vi "周期设置_氨氮.vi"() -> ()   [LabVIEW 2016, in "斯坦道氨氮.lvlib"]
uses:
  <vilib>/Utility/miscctls.llb/LVPointTypeDef.ctl
  <vilib>/Utility/config.llb/NI_LVConfig.lvlib
panel:
  in  "运行周期":T1={"运行模式"=enum."维护模式", "质控频次"=enum."关闭", "空白核查时间"=2, "跨度核查时间"=6, "24H周期设置"=[]} {"跨度核查时间" items=["00H", "01H", "02H", "03H", "04H", "05H", "06H", "07H", "08H", "09H", "10H", "11H", "12H", "13H", "14H", "15H", "16H", "17H", "18H", "19H", "20H", "21H", "22H", "23H", "关闭"]; "空白核查时间" items=["00H", "01H", "02H", "03H", "04H", "05H", "06H", "07H", "08H", "09H", "10H", "11H", "12H", "13H", "14H", "15H", "16H", "17H", "18H", "19H", "20H", "21H", "22H", "23H", "关闭"]}
  # "运行模式："
  # "质控频次："
  # "零点核查时间："
  # "跨度核查时间："
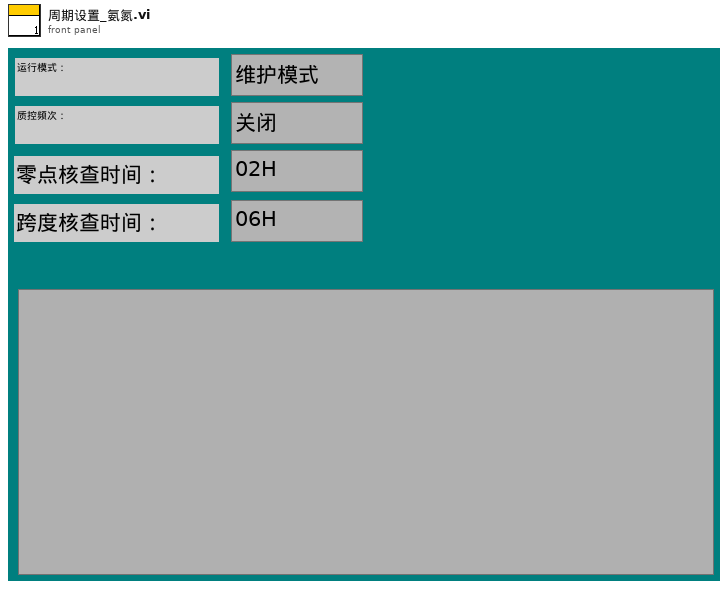
[diagram p1: front panel]
types:
  T1 = cluster{"运行模式":enum16{"维护模式", "常规模式", "应急模式", "质控模式"}, "质控频次":enum16{"关闭", "每天", "星期一", "星期二", "星期三", "星期四", "星期五", "星期六", "星期日"}, "空白核查时间":u16, "跨度核查时间":u16, "24H周期设置":bool[]}
  T2 = typedef "LVPointTypeDef.ctl" = cluster{"Horizontal":i16, "Vertical":i16}
  T3 = enum16{"启动测量", "标样核查", "零点核查", "跨度核查", "空白测试", "平行样测试", "加标回收", "空白校准", "标样校准", "初始化（清洗）", "停止测试", "仪器重启", "校时", "模式设置", "测量间隔设置"}
  T4 = cluster{"系统时间":timestamp, "工作状态":enum16{"空闲", "水样测试", "标样核查", "零点核查", "跨度核查", "空白测试", "平行样测试", "加标回收", "空白校准", "标样校准", "初始化（清洗）"}, "测量模式":enum16{"待机", "连续模式", "周期模式", "定点模式", "受控模式", "手动模式"}, "告警代码":u16, "故障代码":u16, "日志代码":u16, "软件版本":u16, "F0":sgl, "F1":sgl, "F2":sgl, "F3":sgl, "T":sgl, "H":sgl, "id":u16, "flowid":u16, "量程":u16, "总磷控温温度1":sgl, "营养盐控温温度2":sgl, "ADC":sgl}
  T5 = enum16{"关闭", "每天", "星期一", "星期二", "星期三", "星期四", "星期五", "星期六", "星期日"}
  T6 = typedef "LVDateTimeRec.ctl" = cluster{"秒数的小数部分":dbl, "秒":i32, "分":i32, "时":i32, "日":i32, "月":i32, "年":i32, "天数（周）":i32, "天数（年）":i32, "DST":i32}
  T7 = enum32{"Bad", "Idle", "Run top level", "Running"}
  T8 = typedef "NI_LVConfig.lvlib/Config Data RefNum.ctl" = refnum<k1>
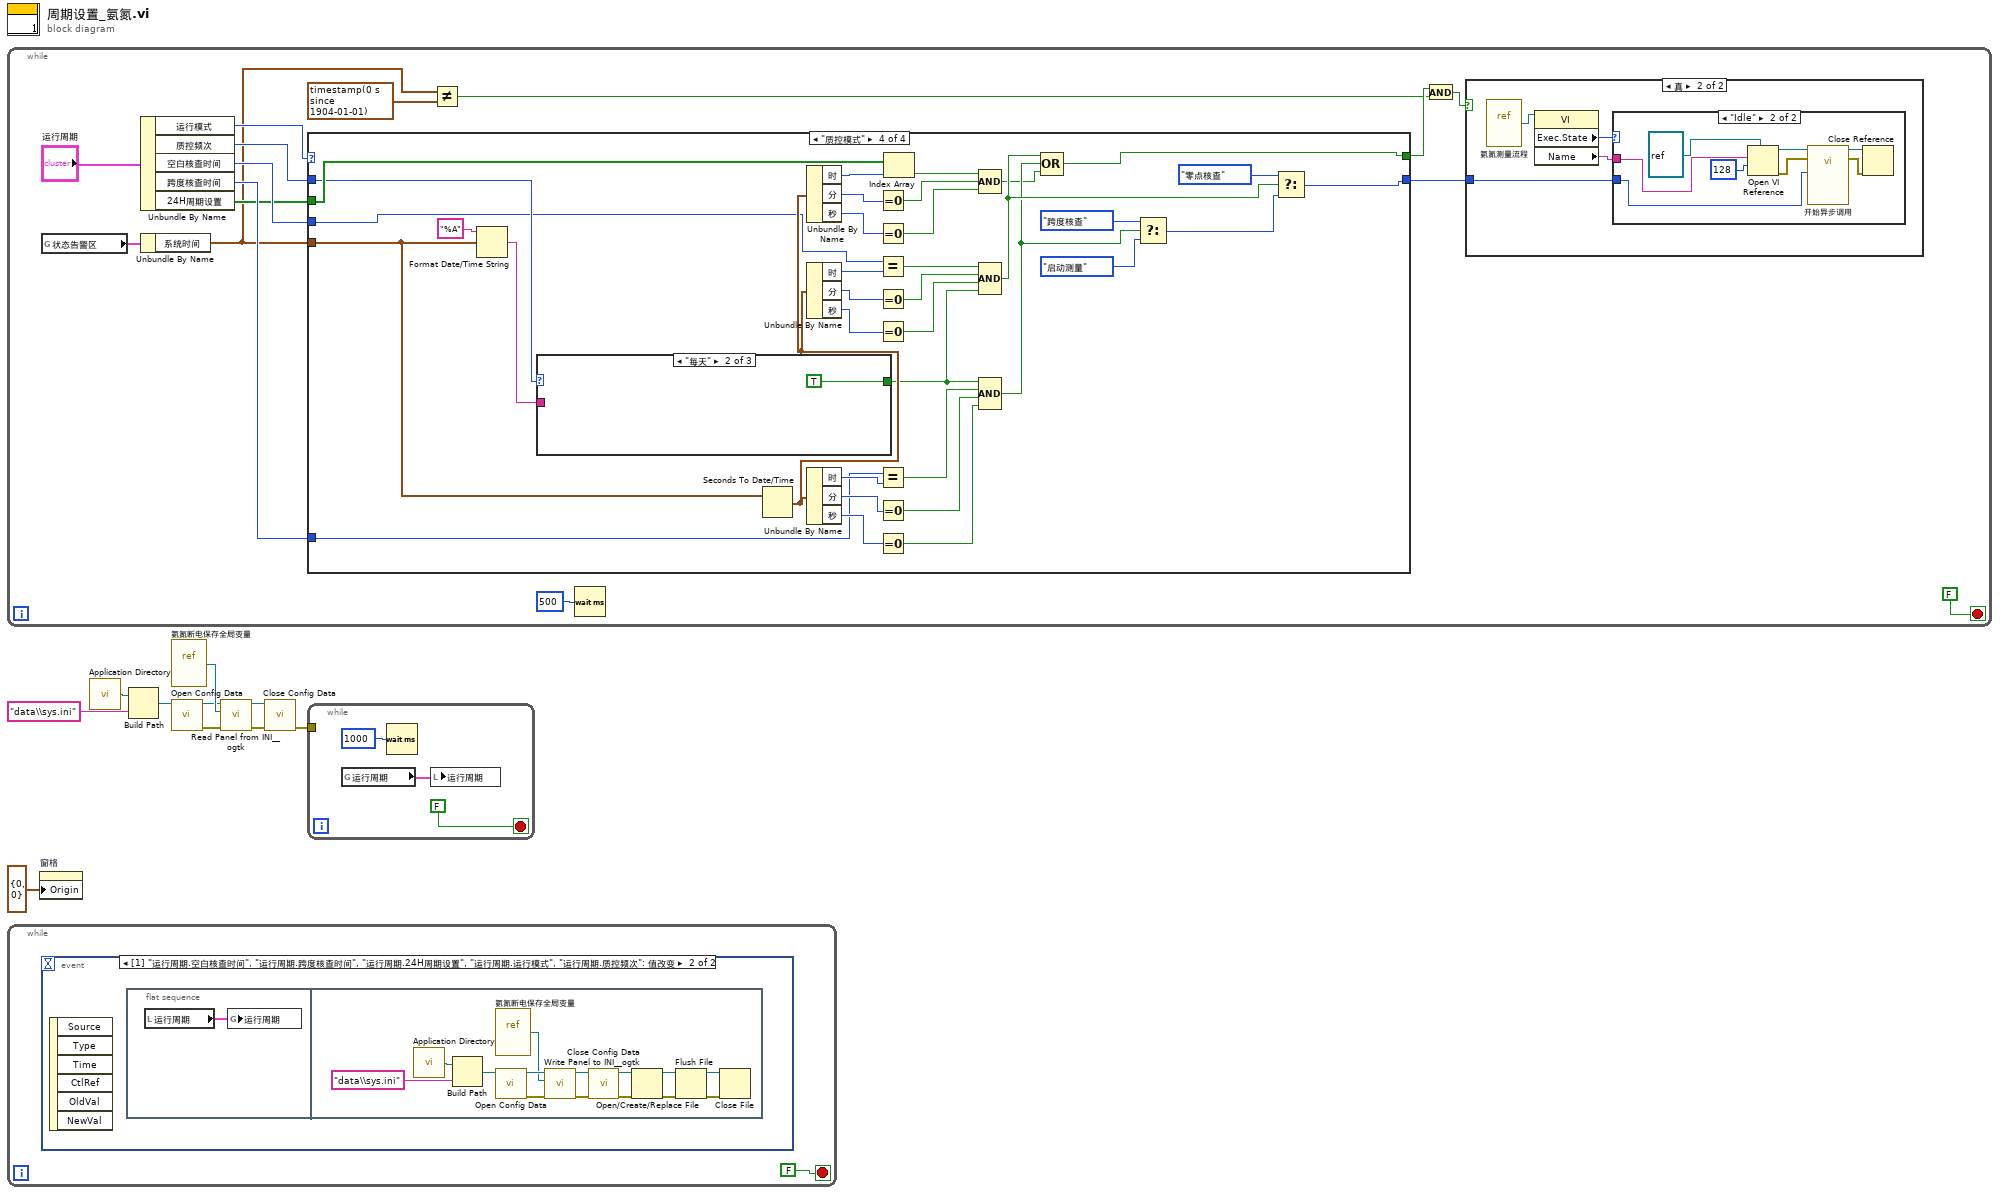
[diagram p0: block diagram]
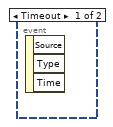
[diagram p2: hidden frame]
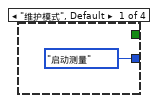
[diagram p5: hidden frame]
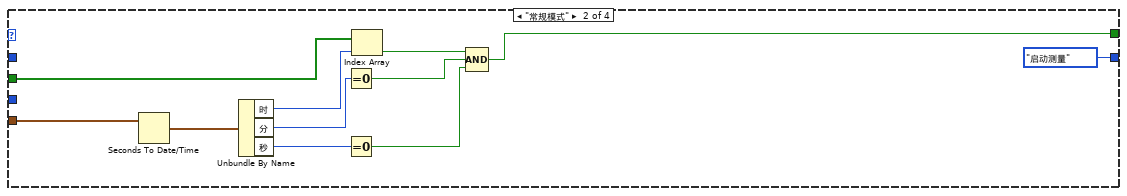
[diagram p6: hidden frame]
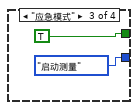
[diagram p7: hidden frame]
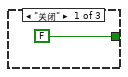
[diagram p8: hidden frame]
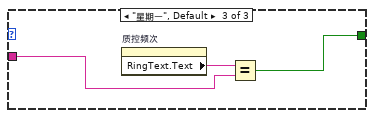
[diagram p9: hidden frame]
diagram:
  n1 = while {
    stop <- FALSE stop-if-true
    n2 = global read "VAR氨氮全局变量.vi" "状态告警区"() -> (w15:T4)
    n3 = Unbundle By Name("运行周期") -> ("运行模式"=w22:enum16{"维护模式", "常规模式", "应急模式", "质控模式"}, "质控频次"=w21:T5, "空白核查时间"=w20:u16, "跨度核查时间"=w19:u16, "24H周期设置"=w18:bool[])
    n4 = Unbundle By Name(w15) -> ("系统时间"=w14:timestamp)
    n5 = case shown="\"质控模式\"" w22 {
      tunnel: w14 -> [_ w49 _ w87]
      tunnel: w18 -> [_ w46 _ w84]
      tunnel: [_ w40 TRUE w64] -> w17
      tunnel: [T3."启动测量" ("控制命令") T3."启动测量" ("控制命令") T3."启动测量" ("控制命令") w60] -> w16
      tunnel: w21 -> [_ _ _ w57]
      tunnel: w20 -> [_ _ _ w56]
      tunnel: w19 -> [_ _ _ w55]
      frame "维护模式", Default {
      }
      frame "常规模式" {
        n6 = Seconds To Date/Time(time stamp (now)=w49) -> (date time rec=w48:T6)  [unwired: 1 in]
        n7 = Unbundle By Name(w48) -> ("时"=w47:i32, "分"=w45:i32, "秒"=w44:i32)
        n8 = Equal To 0?(x=w45) -> (x = 0?=w42:bool)
        n9 = Equal To 0?(x=w44) -> (x = 0?=w41:bool)
        n10 = Index Array(array=w46, index=w47) -> (element=w43:bool)
        n11 = Compound Arithmetic op=AND ("复合运算")(w43, w42, w41) -> (w40:bool)
      }
      frame "应急模式" {
      }
      frame "质控模式" {
        n12 = Format Date/Time String(time format string (%c)="%A" ("时间格式字符串(%c)"), seconds (now)=w87) -> (date/time string=w85:string)  [unwired: 1 in]
        n13 = case shown="\"每天\"" w57 {
          tunnel: w85 -> [_ _ w91]
          tunnel: [FALSE TRUE w90] -> w58
          frame "关闭" {
          }
          frame "每天" {
          }
          frame "星期一", Default {
            n14 = property on="质控频次" class="Enum (严格)"() -> ("RingText.Text"=w92:string)  [unwired: 2 in, 2 out]
            n15 = Equal?(x=w92, y=w91) -> (x = y?=w90:bool)
          }
        }
        n16 = Seconds To Date/Time(time stamp (now)=w87) -> (date time rec=w68:T6)  [unwired: 1 in]
        n17 = Unbundle By Name(w68) -> ("时"=w83:i32, "分"=w81:i32, "秒"=w79:i32)
        n18 = Unbundle By Name(w68) -> ("时"=w77:i32, "分"=w76:i32, "秒"=w75:i32)
        n19 = Unbundle By Name(w68) -> ("时"=w69:i32, "分"=w70:i32, "秒"=w71:i32)
        n20 = Equal To 0?(x=w81) -> (x = 0?=w80:bool)
        n21 = Equal To 0?(x=w79) -> (x = 0?=w78:bool)
        n22 = Equal?(x=w56, y=w77) -> (x = y?=w74:bool)
        n23 = Equal To 0?(x=w76) -> (x = 0?=w73:bool)
        n24 = Equal To 0?(x=w75) -> (x = 0?=w72:bool)
        n25 = Equal?(x=w55, y=w69) -> (x = y?=w67:bool)
        n26 = Equal To 0?(x=w70) -> (x = 0?=w66:bool)
        n27 = Equal To 0?(x=w71) -> (x = 0?=w65:bool)
        n28 = Index Array(array=w84, index=w83) -> (element=w82:bool)
        n29 = Compound Arithmetic op=AND ("复合运算")(w82, w80, w78) -> (w59:bool)
        n30 = Compound Arithmetic op=AND ("复合运算")(w74, w73, w72, w58) -> (w63:bool)
        n31 = Compound Arithmetic op=AND ("复合运算")(w58, w67, w66, w65) -> (w62:bool)
        n32 = Compound Arithmetic op=OR ("复合运算")(w63, w62, w59) -> (w64:bool)
        n33 = Select(t=T3."跨度核查" ("控制命令"), s=w62, f=T3."启动测量" ("控制命令")) -> (s? t:f=w61:T3)
        n34 = Select(t=T3."零点核查" ("控制命令"), s=w63, f=w61) -> (s? t:f=w60:T3)
      }
    }
    n35 = Not Equal?(x=w14, y=timestamp(0 s since 1904-01-01)) -> (x != y?=w11:bool)
    n36 = Wait (ms)(milliseconds to wait=u32 500 ("等待时间（毫秒）")) -> ()  [unwired: 1 out]
    n37 = And(x=w17, y=w11) -> (x .and. y?=w12:bool)
    n38 = case shown="真" w12 {
      tunnel: w16 -> [_ w27]
      frame False {
      }
      frame True {
        n39 = vi-ref "氨氮测量流程.vi"() -> (w28:refnum<vi>)
        n40 = property class="VI"(reference=w28) -> ("Exec.State"=w26:T7, "Name"=w29:string)  [unwired: 1 in, 2 out]
        n41 = case shown="\"Idle\"" w26 {
          tunnel: w29 -> [_ w33]
          tunnel: w27 -> [_ w31]
          frame "Bad", Default {
          }
          frame "Idle" {
            n42 = Open VI Reference(type specifier VI Refnum (for type only)=refnum<vi> refnum, vi path=w33, options=128 ("选项")) -> (vi reference=w34:refnum<vi>, error out=w35:errorcluster)  [unwired: 3 in]
            n43 = call-by-ref "开始异步调用"(reference=w34, error in=w35, "控制命令"=w31) -> (reference out=w36:refnum<vi>, error out=w37:errorcluster)  [unwired: 11 in]
            n44 = Close Reference(reference=w36, error in (no error)=w37) -> ()  [unwired: 1 out]
          }
        }
      }
    }
  }
  n45 = while {
    stop <- FALSE stop-if-true
    n46 = event shown="[1] \"运行周期.空白核查时间\", \"运行周期.跨度核查时间\", \"运行周期.24H周期设置\", \"运行周期.运行模式\", \"运行周期.质控频次\": 值改变" {
      selector: _ -> [_ _]
      dyn-events: _ -> [_ _]
      timeout: _ -> [_ _]
      event Timeout {
        n47 = event-data() -> ()  [unwired: 1 in, 3 out]
      }
      event "运行周期.空白核查时间", "运行周期.跨度核查时间", "运行周期.24H周期设置", "运行周期.运行模式", "运行周期.质控频次": Value Change {
        n48 = event-data() -> ()  [unwired: 1 in, 6 out]
        n49 = flat-sequence {
          frame #0 {
            n50 = local read "运行周期"() -> (w94:T1)
            n51 = global write "氨氮断电保存全局变量.vi" "运行周期"(w94) -> ()
          }
          frame #1 {
            n52 = call <vilib>:"Application Directory.vi"() -> ("Application Directory"=w108:path)
            n53 = Build Path(base path=w108, name or relative path="data\\sys.ini" ("名称或相对路径")) -> (appended path=w106:path)
            n54 = vi-ref "氨氮断电保存全局变量.vi"() -> (w104:refnum<vi>)
            n55 = call <vilib>:"Open Config Data.vi"("configuration file path"=w106) -> ("error out"=w102:errorcluster, "refnum"=w105:T8)  [unwired: 8 in, 1 out]
            n56 = call <userlib>:"Write Panel to INI__ogtk.vi"("error in (no error)"=w102, "VI ref"=w104, "refnum"=w105) -> ("error out"=w101:errorcluster, "refnum out"=w103:T8)  [unwired: 7 in]
            n57 = call <vilib>:"Close Config Data.vi"("error in (no error)"=w101, "refnum"=w103) -> ("error out"=w96:errorcluster, "file path"=w95:path)  [unwired: 8 in]
            n58 = Open/Create/Replace File(file path (use dialog)=w95, error in=w96) -> (refnum out=w99:refnum<file>, error out=w100:errorcluster)  [unwired: 4 in, 1 out]
            n59 = Flush File(refnum=w99, error in=w100) -> (refnum out=w98:refnum<file>, error out=w97:errorcluster)
            n60 = Close File(refnum=w98, error in=w97) -> ()  [unwired: 2 out]
          }
        }
      }
    }
  }
  n61 = property on="窗格" class="Pane"("Origin"=T2 {"Horizontal"=0, "Vertical"=0} ("原点")) -> ()  [unwired: 2 in, 2 out]
  n62 = call <vilib>:"Application Directory.vi"() -> ("Application Directory"=w3:path)
  n63 = Build Path(base path=w3, name or relative path="data\\sys.ini" ("名称或相对路径")) -> (appended path=w5:path)
  n64 = vi-ref "氨氮断电保存全局变量.vi"() -> (w7:refnum<vi>)
  n65 = call <vilib>:"Open Config Data.vi"("configuration file path"=w5) -> ("error out"=w9:errorcluster, "refnum"=w6:T8)  [unwired: 8 in, 1 out]
  n66 = call <userlib>:"Read Panel from INI__ogtk.vi"("error in (no error)"=w9, "VI ref"=w7, "refnum"=w6) -> ("error out"=w10:errorcluster, "refnum out"=w8:T8)  [unwired: 7 in]
  n67 = call <vilib>:"Close Config Data.vi"("error in (no error)"=w10, "refnum"=w8) -> ("error out"=w2:errorcluster)  [unwired: 8 in, 1 out]
  n68 = while {
    tunnel: w2 -> [_]
    stop <- FALSE stop-if-true
    n69 = global read "氨氮断电保存全局变量.vi" "运行周期"() -> (w109:T1)
    n70 = Wait (ms)(milliseconds to wait=u32 1000 ("等待时间（毫秒）")) -> ()  [unwired: 1 out]
    n71 = local write "运行周期"(w109) -> ()
  }
